vi "rawTime2ProperTime.vi"(2 "Tdchhit time":i64, 3 "Init":bool) -> (0 "32ps res unsigned":u64, 1 "Added time":u64)   [LabVIEW 2016, in "HPTDC Driver Library.lvlib"]
uses:
  HPTDC Driver Library Folder/HPTDC Driver Library.lvlib
  Global Variables/Global Resolution.vi
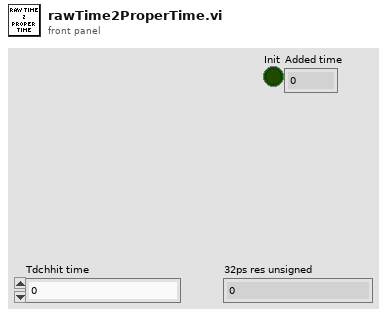
[diagram p1: front panel]
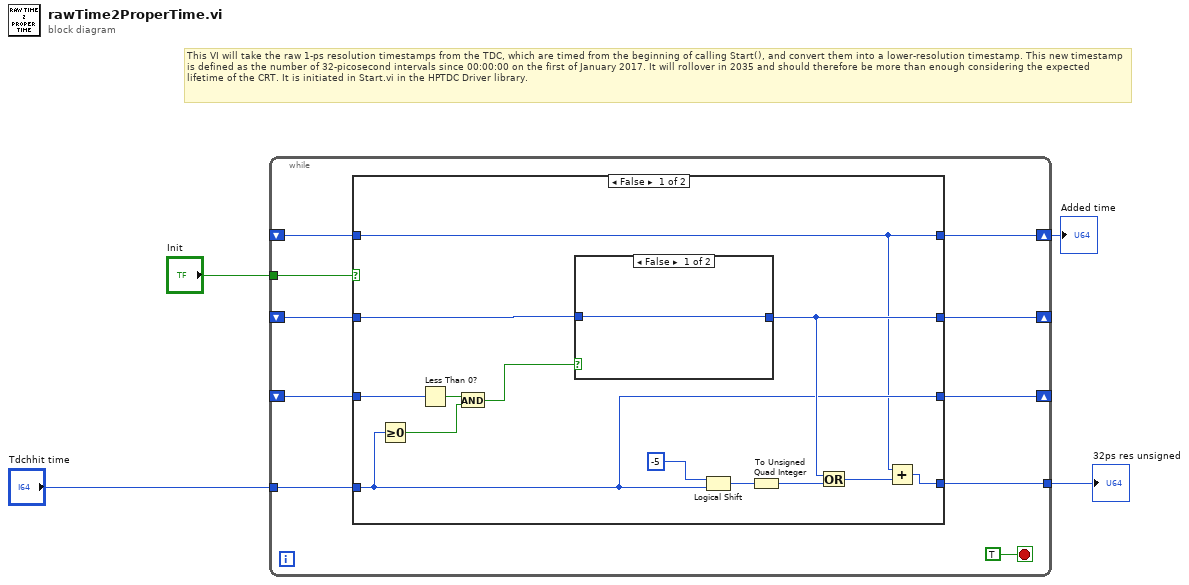
[diagram p0: block diagram]
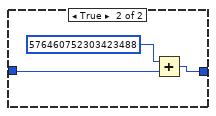
[diagram p2: hidden frame]
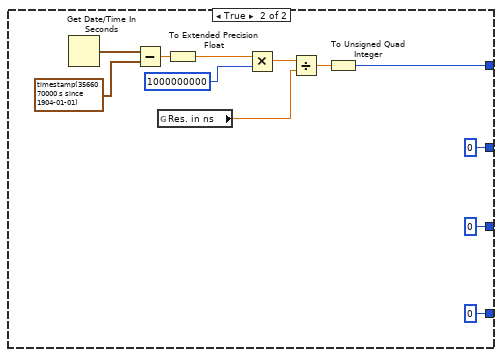
[diagram p3: hidden frame]
diagram:
  # "This VI will take the raw 1-ps resolution timestamps from the TDC, which are timed from the beginning of calling Start(), and convert them into a lower-resolution timestamp. This new timestamp is defined as the number of 32-picosecond intervals since 00:00:00 on the first of January 2017. It will rollover in 2035 and should therefore be more than enough considering the expected lifetime of the CRT. It is initiated in Start.vi in the HPTDC Driver library."
  n1 = while {
    tunnel: "Tdchhit time" -> [w12]
    tunnel: [w9] -> w4
    shift-right: [w7] -> _
    shift-left: _ -> [w13]
    shift-right: [w10] -> _
    shift-left: _ -> [w11]
    tunnel: "Init" -> [w8]
    shift-right: [w6] -> w1
    shift-left: _ -> [w5]
    stop <- TRUE stop-if-true
    n2 = case shown="False" w8 {
      tunnel: w13 -> [w25 _]
      tunnel: w12 -> [w18 _]
      tunnel: w11 -> [w21 _]
      tunnel: [w19 u64 0] -> w10
      tunnel: [w16 u64 0] -> w9
      tunnel: [w18 i64 0 ("Tdchhit time")] -> w7
      tunnel: [w15 w32] -> w6
      tunnel: w5 -> [w15 _]
      frame False {
        n3 = Greater Or Equal To 0?(x=w18) -> (x >= 0?=w23:bool)
        n4 = Less Than 0?(x=w25) -> (x < 0?=w24:bool)
        n5 = And(x=w24, y=w23) -> (x .and. y?=w22:bool)
        n6 = case shown="False" w22 {
          tunnel: w21 -> [w28 w30]
          tunnel: [w28 w29] -> w19
          frame False {
          }
          frame True {
            n7 = Add(x=u64 576460752303423488, y=w30) -> (x+y=w29:u64)
          }
        }
        n8 = Logical Shift(y=i16 -5, x=w18) -> (x << y=w26:i64)
        n9 = To Unsigned Quad Integer(1:w26) -> (0:w20:u64)
        n10 = Or(x=w19, y=w20) -> (x .or. y?=w17:u64)
        n11 = Add(x=w15, y=w17) -> (x+y=w16:u64)
      }
      frame True {
        n12 = Get Date/Time In Seconds() -> (seconds since 1Jan1904=w40:timestamp)
        n13 = Subtract(x=w40, y=timestamp(3566070000 s since 1904-01-01)) -> (x-y=w37:dbl)
        n14 = global read "Global Resolution.vi" "Res. in ns"() -> (w34:ext)
        n15 = To Extended Precision Float(1:w37) -> (0:w36:ext)
        n16 = Multiply(x=w36, y=1000000000) -> (x*y=w35:ext)
        n17 = Divide(x=w35, y=w34) -> (x/y=w33:ext)
        n18 = To Unsigned Quad Integer(1:w33) -> (0:w32:u64)
      }
    }
  }
  "32ps res unsigned" <- w4
  "Added time" <- w1
